vi "Compare Controller Type.vi"(6 "Raise error? (F)":bool, 8 "error in (no error)":errorcluster, 10 "Controller Type":T1, 11 "Generic Controller in":refnum<class "Generic Plugin.lvclass">) -> (0 "error out":errorcluster, 2 "Match?":bool, 3 "Generic Controller out":refnum<class "Generic Plugin.lvclass">)   [LabVIEW 2020, in "Generic Plugin.lvclass"]
uses:
  Generic Plugin.lvclass
  Controller Type.ctl
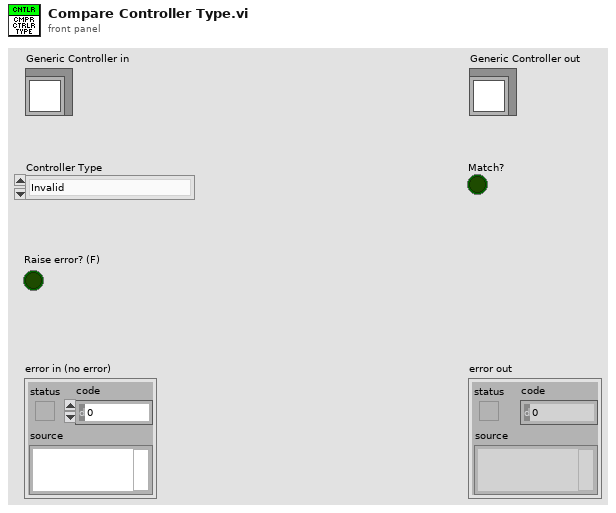
[diagram p1: front panel]
types:
  T1 = typedef "Generic Plugin.lvclass/Controller Type.ctl" = enum16{"Invalid", "Temperature Controller", "Pump Controller", "Generic Optimizer", "LC Parser"}
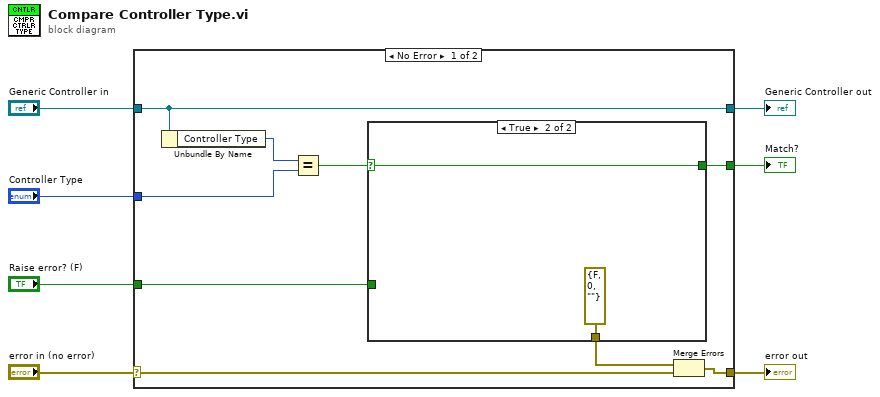
[diagram p0: block diagram]
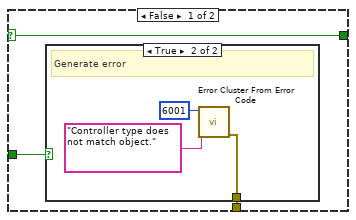
[diagram p2: hidden frame]
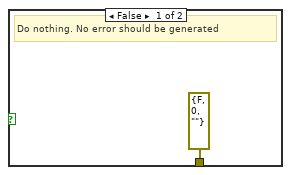
[diagram p3: hidden frame]
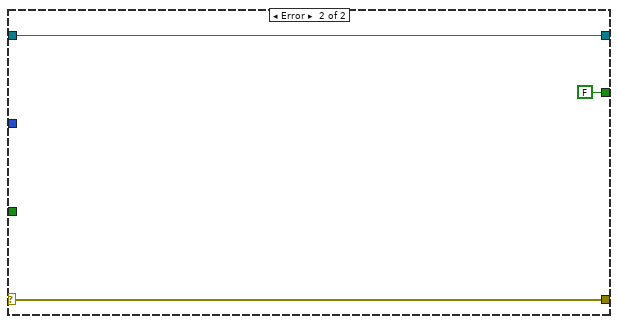
[diagram p4: hidden frame]
diagram:
  n1 = case shown="No Error" "error in (no error)" {
    selector: "error in (no error)" -> [w16 w28]
    tunnel: [w9 w28] -> w6
    tunnel: [w15 w27] -> w4
    tunnel: "Generic Controller in" -> [w15 w27]
    tunnel: "Controller Type" -> [w14 _]
    tunnel: "Raise error? (F)" -> [w12 _]
    tunnel: [w10 FALSE] -> w1
    frame No Error {
      n2 = Unbundle By Name(w15) -> ("Controller Type"=w13:T1)
      n3 = Equal?(x=w13, y=w14) -> (x = y?=w11:bool)
      n4 = case shown="True" w11 {
        selector: w11 -> [w18 w25]
        tunnel: w12 -> [w19 _]
        tunnel: [w18 w25] -> w10
        tunnel: [w17 errorcluster {"status"=FALSE, "code"=0, "source"=""} ("error out")] -> w8
        frame False {
          n5 = case shown="True" w19 {
            tunnel: [errorcluster {"status"=FALSE, "code"=0, "source"=""} ("error out") w21] -> w17
            frame False {
              # "Do nothing. No error should be generated"
            }
            frame True {
              # "Generate error"
              n6 = call <vilib>:"Error Cluster From Error Code.vi"("error message (\"\")"="Controller type does not match object." ("error message (\"\")"), "error code (0)"=6001) -> ("error out"=w21:errorcluster)  [unwired: 7 in]
            }
          }
        }
        frame True {
        }
      }
      n7 = Merge Errors(w8, w16) -> (w9:errorcluster)
    }
    frame Error {
    }
  }
  "error out" <- w6
  "Generic Controller out" <- w4
  "Match?" <- w1
